vi "Meas Result Get Sweep Data.vi"(6 "equ connection override":T1=enum."Rs-Xs", 8 "freq filter (NaN: no filter)":dbl=nan, 9 "uncertainty mode":T2, 10 "phase index (default: 0)":i32, 11 "result":T5) -> (0 "quantities":T3, 2 "unc(data)":T4, 3 "data":T4)   [LabVIEW 2020]
doc: "Processes collected readings into sweep with uncertainties in selected mode."
uses:
  Meas Results Sweep Data.ctl
  Meas Results.ctl
  bridge/Bridge Frequency Readings Data.ctl
  drivers/TWM client/Meas Proc QWTB Spectrum Data.ctl
  drivers/TWM client/TWM Phase Info.ctl
  Meas Quantity Names.ctl
  Meas Results Sweep Data Uncertainty Mode.ctl
  Impedance Equivalent Circuit.ctl
  varilib/varilib.lvlib
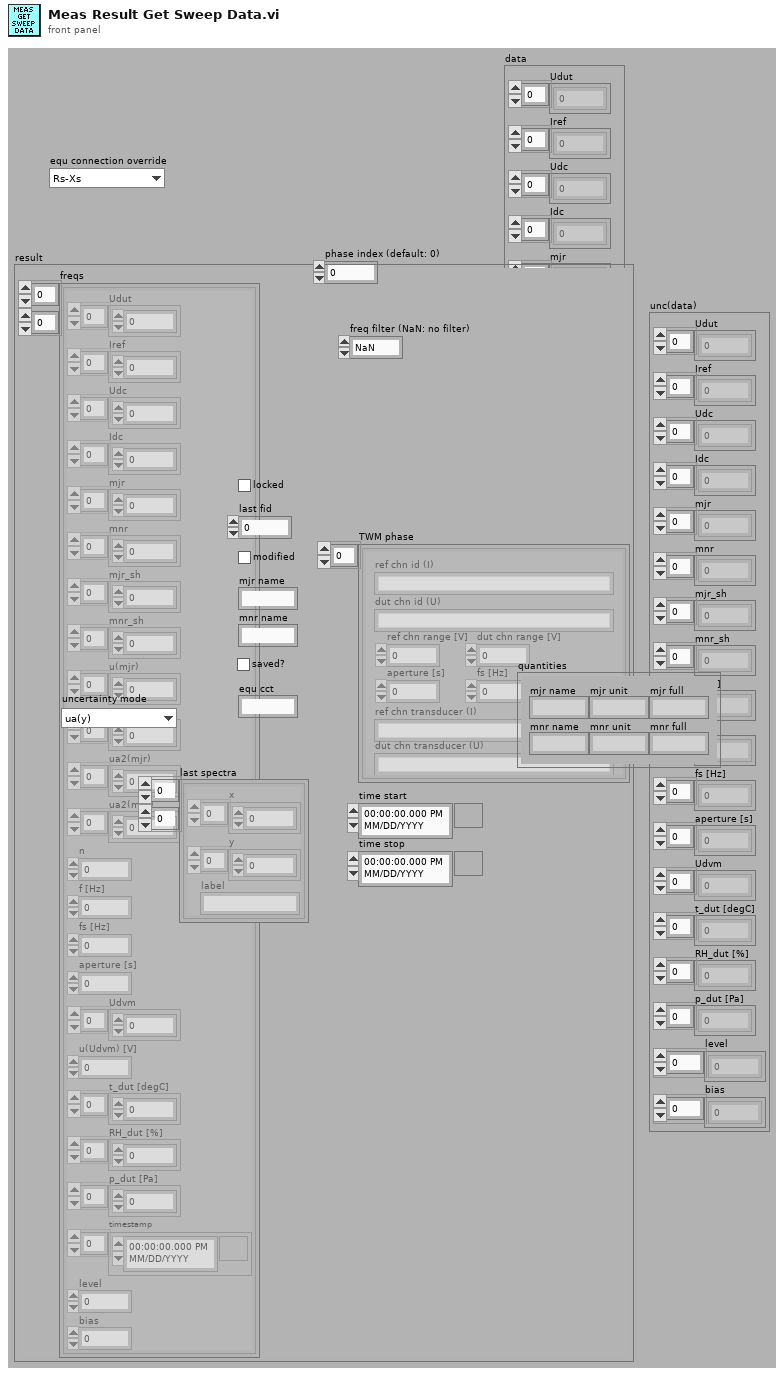
[diagram p1: front panel]
types:
  T1 = typedef "Impedance Equivalent Circuit.ctl" = enum16{"Keep original", "Rs-Xs", "Gp-Bp", "Z-phid", "Z-phir", "Y-phid", "Y-phir", "Cp-D", "Cp-Q", "Cp-Rp", "Cp-Gp", "Cs-D", "Cs-Q", "Cs-Rs", "Ls-Rs", "Ls-Q", "Rs-Tau"}
  T2 = typedef "Meas Results Sweep Data Uncertainty Mode.ctl" = enum16{"ua(y)", "ua(y) (p=95%)", "uc(y) (p=95%)"}
  T3 = typedef "Meas Quantity Names.ctl" = cluster{"mjr name":string, "mnr name":string, "mjr unit":string, "mnr unit":string, "mjr full":string, "mnr full":string}
  T4 = typedef "Meas Results Sweep Data.ctl" = cluster{"Udut":dbl[], "Iref":dbl[], "Udc":dbl[], "Idc":dbl[], "mjr":dbl[], "mnr":dbl[], "mjr_sh":dbl[], "mnr_sh":dbl[], "f [Hz]":dbl[], "n [-]":i32[], "fs [Hz]":dbl[], "aperture [s]":dbl[], "Udvm":dbl[], "t_dut [degC]":dbl[], "RH_dut [%]":dbl[], "p_dut [Pa]":dbl[], "level":dbl[], "bias":dbl[]}
  T5 = typedef "Meas Results.ctl" = cluster{"freqs":T6[][], "locked":bool, "last fid":i32, "modified":bool, "mjr name":string, "mnr name":string, "last spectra":T7[][], "saved?":bool, "TWM phase":T8[], "time start":timestamp, "time stop":timestamp, "equ cct":string}
  T6 = typedef "Bridge Frequency Readings Data.ctl" = cluster{"Udut":dbl[], "Iref":dbl[], "Udc":dbl[], "Idc":dbl[], "mjr":dbl[], "mnr":dbl[], "mjr_sh":dbl[], "mnr_sh":dbl[], "u(mjr)":dbl[], "u(mnr)":dbl[], "ua2(mjr)":dbl[], "ua2(mnr)":dbl[], "n":i32, "f [Hz]":dbl, "fs [Hz]":dbl, "aperture [s]":dbl, "Udvm":dbl[], "u(Udvm) [V]":dbl, "t_dut [degC]":dbl[], "RH_dut [%]":dbl[], "p_dut [Pa]":dbl[], "timestamp":timestamp[], "level":dbl, "bias":dbl}
  T7 = typedef "Meas Proc QWTB Spectrum Data.ctl" = cluster{"x":sgl[], "y":sgl[], "label":string}
  T8 = typedef "TWM Phase Info.ctl" = cluster{"ref chn id (I)":string, "dut chn id (U)":string, "ref chn range [V]":dbl, "dut chn range [V]":dbl, "aperture [s]":dbl, "fs [Hz]":dbl, "ref chn transducer (I)":string, "dut chn transducer (U)":string}
  T9 = typedef "Impedance Equivalent Circuit Type Info.ctl" = cluster{"major":string, "major unit":string, "minor":string, "minor unit":string, "combined":string, "major+unit":string, "minor+unit":string}
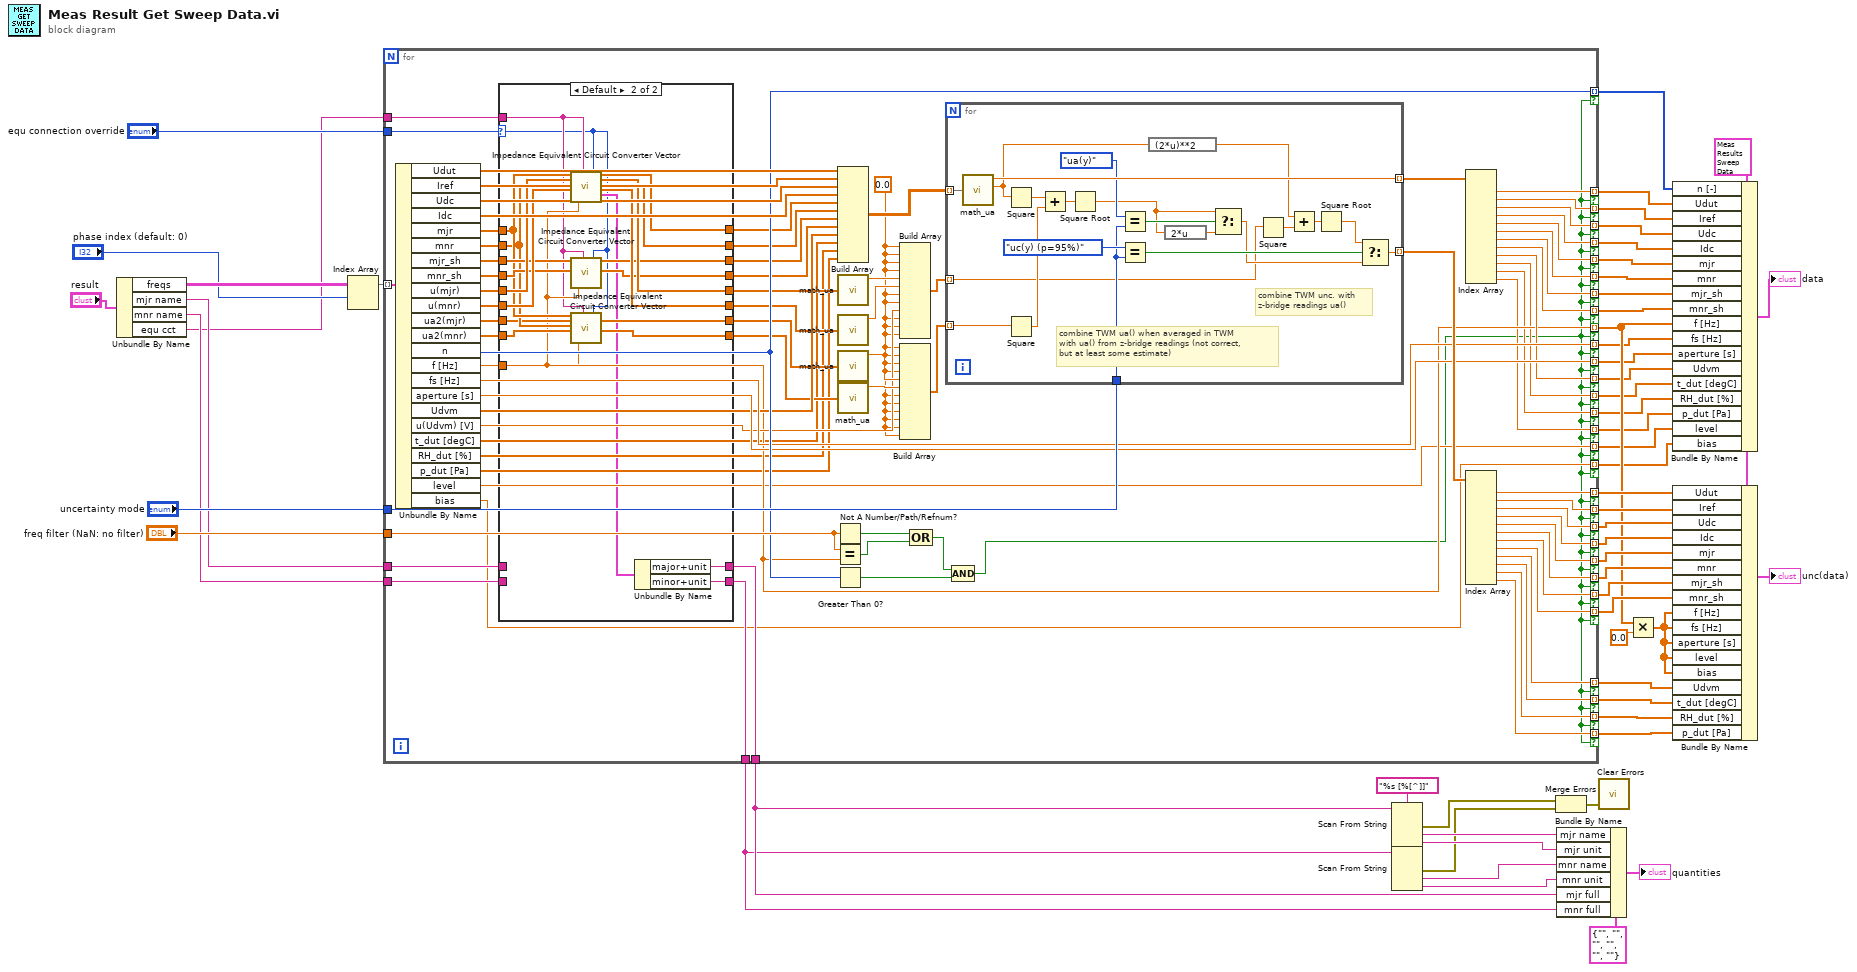
[diagram p0: block diagram]
diagram:
  w36 = "%s [%[^]]" ("format string")
  w42 = T4 {"Udut"=[], "Iref"=[], "Udc"=[], "Idc"=[], "mjr"=[], "mnr"=[], "mjr_sh"=[], "mnr_sh"=[], "f [Hz]"=[], "n [-]"=[], "fs [Hz]"=[], "aperture [s]"=[], "Udvm"=[], "t_dut [degC]"=[], "RH_dut [%]"=[], "p_dut [Pa]"=[], "level"=[], "bias"=[]} ("data")
  n1 = Unbundle By Name("result") -> ("freqs"=w56:T6[][], "mjr name"=w13:string, "mnr name"=w14:string, "equ cct"=w10:string)
  n2 = Index Array(array=w56, index (row)="phase index (default: 0)") -> (element=w24:T6[])  [unwired: 1 in]
  n3 = for {
    tunnel: w24 -> [w136] mode=indexing
    tunnel: [w129] -> w55 mode=indexing if=w58
    tunnel: [w128] -> w54 mode=indexing if=w58
    tunnel: [w127] -> w53 mode=indexing if=w58
    tunnel: [w126] -> w52 mode=indexing if=w58
    tunnel: [w125] -> w51 mode=indexing if=w58
    tunnel: [w124] -> w50 mode=indexing if=w58
    tunnel: [w76] -> w20 mode=indexing if=w58
    tunnel: [w122] -> w49 mode=indexing if=w58
    tunnel: [w121] -> w48 mode=indexing if=w58
    tunnel: [w120] -> w47 mode=indexing if=w58
    tunnel: [w119] -> w46 mode=indexing if=w58
    tunnel: [w118] -> w45 mode=indexing if=w58
    tunnel: [w117] -> w44 mode=indexing if=w58
    tunnel: "uncertainty mode" -> [w110]
    tunnel: [w109] -> w28 mode=indexing if=w58
    tunnel: [w108] -> w27 mode=indexing if=w58
    tunnel: [w107] -> w26 mode=indexing if=w58
    tunnel: [w106] -> w25 mode=indexing if=w58
    tunnel: "freq filter (NaN: no filter)" -> [w105]
    tunnel: [w100] -> w21 mode=indexing if=w58
    tunnel: [w99] -> w19 mode=indexing if=w58
    tunnel: [w98] -> w18 mode=indexing if=w58
    tunnel: [w96] -> w17 mode=indexing if=w58
    tunnel: [w95] -> w16 mode=indexing if=w58
    tunnel: "equ connection override" -> [w71]
    tunnel: w10 -> [w77]
    tunnel: w13 -> [w75]
    tunnel: w14 -> [w74]
    tunnel: [w73] -> w12
    tunnel: [w72] -> w11
    tunnel: [w66] -> w9 mode=indexing if=w58
    tunnel: [w65] -> w8 mode=indexing if=w58
    tunnel: [w64] -> w7 mode=indexing if=w58
    tunnel: [w63] -> w6 mode=indexing if=w58
    tunnel: [w62] -> w5 mode=indexing if=w58
    tunnel: [w61] -> w4 mode=indexing if=w58
    tunnel: [w60] -> w3 mode=indexing if=w58
    tunnel: [w59] -> w2 mode=indexing if=w58
    w67 = 0.0
    n4 = Unbundle By Name(w136) -> ("Udut"=w135:dbl[], "Iref"=w134:dbl[], "Udc"=w133:dbl[], "Idc"=w132:dbl[], "mjr"=w93:dbl[], "mnr"=w91:dbl[], "mjr_sh"=w89:dbl[], "mnr_sh"=w87:dbl[], "u(mjr)"=w85:dbl[], "u(mnr)"=w83:dbl[], "ua2(mjr)"=w81:dbl[], "ua2(mnr)"=w79:dbl[], "n"=w100:i32, "f [Hz]"=w76:dbl, "fs [Hz]"=w99:dbl, "aperture [s]"=w98:dbl, "Udvm"=w97:dbl[], "u(Udvm) [V]"=w94:dbl, "t_dut [degC]"=w70:dbl[], "RH_dut [%]"=w69:dbl[], "p_dut [Pa]"=w68:dbl[], "level"=w60:dbl, "bias"=w59:dbl)
    n5 = case shown="Default" w71 {
      selector: w71 -> [_ w147]
      tunnel: [w146 w166] -> w92
      tunnel: w93 -> [w146 w158]
      tunnel: [w145 w165] -> w90
      tunnel: w91 -> [w145 w157]
      tunnel: [w144 w160] -> w88
      tunnel: w89 -> [w144 w162]
      tunnel: [w143 w159] -> w86
      tunnel: w87 -> [w143 w161]
      tunnel: [w142 w164] -> w84
      tunnel: w85 -> [w142 w168]
      tunnel: [w141 w163] -> w82
      tunnel: w83 -> [w141 w167]
      tunnel: [w140 w154] -> w80
      tunnel: w81 -> [w140 w156]
      tunnel: [w139 w153] -> w78
      tunnel: w79 -> [w139 w155]
      tunnel: w77 -> [_ w151]
      tunnel: w76 -> [_ w152]
      tunnel: [w138 w149] -> w73
      tunnel: [w137 w148] -> w72
      tunnel: w75 -> [w138 _]
      tunnel: w74 -> [w137 _]
      frame "Keep original" {
      }
      frame Default {
        n6 = call "Impedance Equivalent Circuit Converter Vector.vi"("major in"=w158, "u(major) in"=w168, "minor in"=w157, "u(minor) in"=w167, "f scalar [Hz]"=w152, "type in by string"=w151, "type out"=w147) -> ("major out"=w166:dbl[], "u(major) out"=w164:dbl[], "minor out"=w165:dbl[], "u(minor) out"=w163:dbl[], "type out info"=w150:T9)  [unwired: 7 in, 1 out]
        n7 = call "Impedance Equivalent Circuit Converter Vector.vi"("major in"=w162, "minor in"=w161, "f scalar [Hz]"=w152, "type in by string"=w151, "type out"=w147) -> ("major out"=w160:dbl[], "minor out"=w159:dbl[])  [unwired: 9 in, 4 out]
        n8 = call "Impedance Equivalent Circuit Converter Vector.vi"("major in"=w158, "u(major) in"=w156, "minor in"=w157, "u(minor) in"=w155, "f scalar [Hz]"=w152, "type in by string"=w151, "type out"=w147) -> ("u(major) out"=w154:dbl[], "u(minor) out"=w153:dbl[])  [unwired: 7 in, 4 out]
        n9 = Unbundle By Name(w150) -> ("major+unit"=w149:string, "minor+unit"=w148:string)
      }
    }
    n10 = Not A Number/Path/Refnum?(number/path/refnum=w105) -> (NaN/Path/Refnum?=w104:bool)
    n11 = Equal?(x=w105, y=w76) -> (x = y?=w103:bool)
    n12 = Greater Than 0?(x=w100) -> (x > 0?=w102:bool)
    n13 = Build Array(w135, w134, w133, w132, w92, w90, w88, w86, w97, w70, w69, w68) -> (w131:dbl[][])
    n14 = call "math_ua.vi"("x"=w84) -> ("mean(x)"=w116:dbl)  [unwired: 3 out]
    n15 = call "math_ua.vi"("x"=w82) -> ("mean(x)"=w115:dbl)  [unwired: 3 out]
    n16 = call "math_ua.vi"("x"=w80) -> ("mean(x)"=w114:dbl)  [unwired: 3 out]
    n17 = call "math_ua.vi"("x"=w78) -> ("mean(x)"=w113:dbl)  [unwired: 3 out]
    n18 = Build Array(w67, w67, w67, w67, w116, w115, w67, w67, w94, w67, w67, w67) -> (w112:dbl[])
    n19 = Build Array(w67, w67, w67, w67, w114, w113, w67, w67, w67, w67, w67, w67) -> (w111:dbl[])
    n20 = Compound Arithmetic op=OR(w104, w103) -> (w101:bool)
    n21 = for {
      tunnel: w131 -> [w169] mode=indexing
      tunnel: [w189] -> w130 mode=indexing
      tunnel: [w176] -> w123 mode=indexing
      tunnel: w112 -> [w174] mode=indexing
      tunnel: w111 -> [w188] mode=indexing
      tunnel: w110 -> [w181]
      # "combine TWM ua() when averaged in TWM\nwith ua() from z-bridge readings (not correct,\nbut at least some estimate)"
      # "combine TWM unc. with\nz-bridge readings ua()"
      n22 = call "math_ua.vi"("x"=w169) -> ("mean(x)"=w189:dbl, "ua(x)"=w175:dbl)  [unwired: 2 out]
      n23 = Square(x=w175) -> (x^2=w187:dbl)
      n24 = Square(x=w188) -> (x^2=w186:dbl)
      n25 = Add(x=w187, y=w186) -> (x+y=w185:dbl)
      n26 = Square Root(x=w185) -> (sqrt(x)=w178:dbl)
      n27 = Equal?(x=Meas_Results_Sweep_Data_Uncertainty_Mode."ua(y)", y=w181) -> (x = y?=w182:bool)
      n28 = Equal?(x=Meas_Results_Sweep_Data_Uncertainty_Mode."uc(y) (p=95%)", y=w181) -> (x = y?=w184:bool)
      n29 = expression code="(2*u)**2"(w175) -> (w172:dbl)
      n30 = expression code="2*u"(w178) -> (w177:dbl)
      n31 = Select(t=w178, s=w182, f=w177) -> (s? t:f=w179:dbl)
      n32 = Square(x=w174) -> (x^2=w173:dbl)
      n33 = Add(x=w172, y=w173) -> (x+y=w171:dbl)
      n34 = Square Root(x=w171) -> (sqrt(x)=w170:dbl)
      n35 = Select(t=w170, s=w184, f=w179) -> (s? t:f=w176:dbl)
    }
    n36 = Compound Arithmetic op=AND(w101, w102) -> (w58:bool)
    n37 = Index Array(array=w130) -> (element #1=w129:dbl, element #2=w128:dbl, element #3=w127:dbl, element #4=w126:dbl, element #5=w125:dbl, element #6=w124:dbl, element #7=w109:dbl, element #8=w108:dbl, element #9=w96:dbl, element #10=w66:dbl, element #11=w65:dbl, element #12=w64:dbl)  [unwired: 12 in]
    n38 = Index Array(array=w123) -> (element #1=w122:dbl, element #2=w121:dbl, element #3=w120:dbl, element #4=w119:dbl, element #5=w118:dbl, element #6=w117:dbl, element #7=w107:dbl, element #8=w106:dbl, element #9=w95:dbl, element #10=w63:dbl, element #11=w62:dbl, element #12=w61:dbl)  [unwired: 12 in]
  }
  n39 = Scan From String(format string=w36, input string=w12) -> (error out=w31:errorcluster, output 1=w38:string, output 2=w37:string)  [unwired: 4 in, 2 out]
  n40 = Scan From String(format string=w36, input string=w11) -> (error out=w32:errorcluster, output 1=w35:string, output 2=w34:string)  [unwired: 4 in, 2 out]
  n41 = Merge Errors(w31, w32) -> (w30:errorcluster)
  n42 = Bundle By Name(cluster=T3 {"mjr name"="", "mnr name"="", "mjr unit"="", "mnr unit"="", "mjr full"="", "mnr full"=""} ("quantities"), "mjr name"=w38, "mjr unit"=w37, "mnr name"=w35, "mnr unit"=w34, "mjr full"=w12, "mnr full"=w11) -> (→"quantities":T3)
  n43 = call <vilib>:"Clear Errors.vi"("error in (no error)"=w30) -> ()  [unwired: 5 in, 2 out]
  n44 = Multiply(x=w20, y=0.0) -> (x*y=w1:dbl[])
  n45 = Bundle By Name(cluster=w42, "n [-]"=w21, "Udut"=w55, "Iref"=w54, "Udc"=w53, "Idc"=w52, "mjr"=w51, "mnr"=w50, "mjr_sh"=w28, "mnr_sh"=w27, "f [Hz]"=w20, "fs [Hz]"=w19, "aperture [s]"=w18, "Udvm"=w17, "t_dut [degC]"=w9, "RH_dut [%]"=w8, "p_dut [Pa]"=w7, "level"=w3, "bias"=w2) -> (→"data":T4)
  n46 = Bundle By Name(cluster=w42, "Udut"=w49, "Iref"=w48, "Udc"=w47, "Idc"=w46, "mjr"=w45, "mnr"=w44, "mjr_sh"=w26, "mnr_sh"=w25, "f [Hz]"=w1, "fs [Hz]"=w1, "aperture [s]"=w1, "level"=w1, "bias"=w1, "Udvm"=w16, "t_dut [degC]"=w6, "RH_dut [%]"=w5, "p_dut [Pa]"=w4) -> (→"unc(data)":T4)
